vi "shutter.vi"(7 "converter box version":i16=1 min=1 max=2, 11 "open?":bool) -> ()   [LabVIEW 2010]
uses:
  <vilib>/eio/EIONode/EIONode.xnode
  <vilib>/rvi/eio/nirviEIOImplementation/nirviEIOImplementation.xnode
  <vilib>/rvi/eio/common/nirviEmuClasses.ctl
  <vilib>/rvi/eio/common/nirviEmuTemplateMethod_noerrors.vi
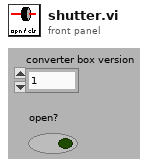
[diagram p1: front panel]
types:
  T1 = typedef "nirviEmuClasses.ctl" = enum16{"IO Read", "IO Write", "Method", "Property Read", "Property Write"}
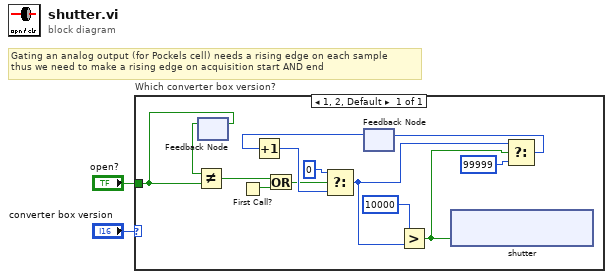
[diagram p0: block diagram]
diagram:
  # "Gating an analog output (for Pockels cell) needs a rising edge on each sample\nthus we need to make a rising edge on acquisition start AND end"
  n1 = case "Which converter box version?" shown="1, 2, Default" "converter box version" {
    tunnel: "open?" -> [w14]
    frame 1, 2, Default {
      n2 = feedback-in #1(w14) -> ()
      n3 = feedback #1() -> (w15:bool)  [unwired: 1 in]
      n4 = Not Equal?(x=w15, y=w14) -> (x != y?=w4:bool)
      n5 = First Call?() -> (First Call?: T/F=w5:bool)
      n6 = Or(x=w4, y=w5) -> (x .or. y?=w3:bool)
      n7 = feedback #2() -> (w12:u32)  [unwired: 1 in]
      n8 = Increment(x=w12) -> (x+1=w11:u32)
      n9 = Select(t=u32 0, s=w3, f=w11) -> (s? t:f=w6:u32)
      n10 = Greater?(x=u32 10000, y=w6) -> (0:w8:bool)
      n11 = xnode "shutter"("Connector0/DIO32"=w8) -> ()  [unwired: 1 in, 1 out]
      n12 = Select(t=w6, s=w8, f=u32 99999) -> (s? t:f=w10:u32)
      n13 = feedback-in #2(w10) -> ()
    }
  }
